vi "returnState.vi"(6 "error IN":errorcluster, 8 "String IN":string) -> (0 "error out":errorcluster, 1 "Return State":T2(ring), 3 "output cluster":T1)   [LabVIEW 2017]
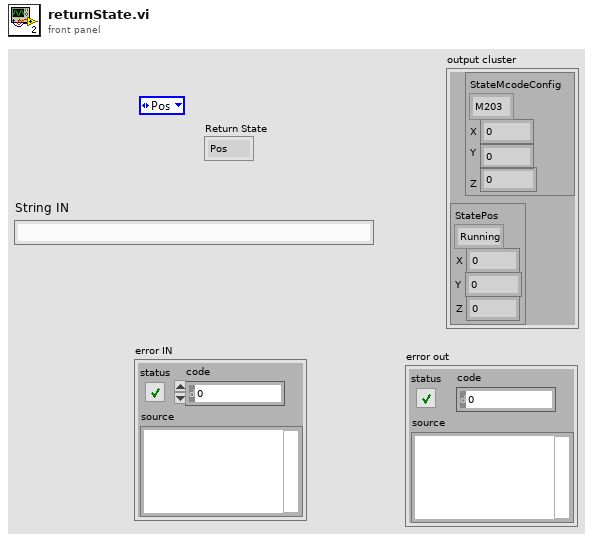
[diagram p1: front panel]
types:
  T1 = cluster{"OUTCONFIG":cluster{"StateMcodeConfig":enum16{"M203", "M201", "M92", "M3001"}, "X":dbl, "Y":dbl, "Z":dbl}, "outPOS":cluster{"StatePos":enum16{"Running", "Waiting", "Pos", "IDLE"}, "X":dbl, "Z":dbl, "Y":dbl}}
  T2 = enum16{"Pos", "Config", "Data1", "Data2", "Step"}
  T3 = cluster{"Enum":enum16{"Running", "Waiting", "Pos", "IDLE"}, dbl, dbl, dbl}
  T4 = cluster{"StateMcodeConfig":enum16{"M203", "M201", "M92", "M3001"}, dbl, dbl, dbl}
  T5 = cluster{cluster{"StateMcodeConfig":enum16{"M203", "M201", "M92", "M3001"}, dbl, dbl, dbl}, cluster{"Enum":enum16{"Running", "Waiting", "Pos", "IDLE"}, dbl, dbl, dbl}}
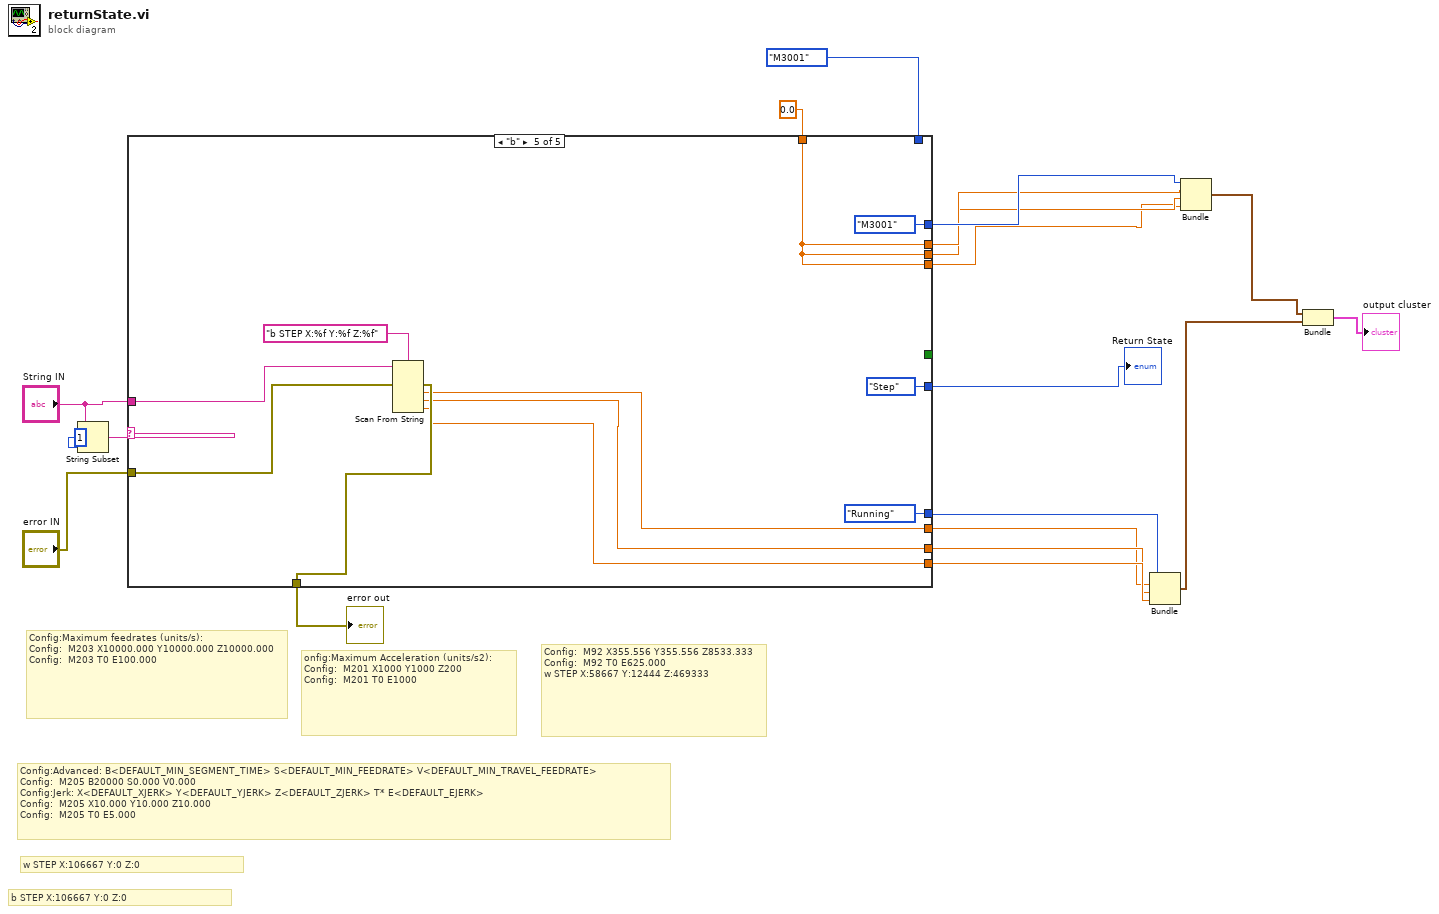
[diagram p0: block diagram]
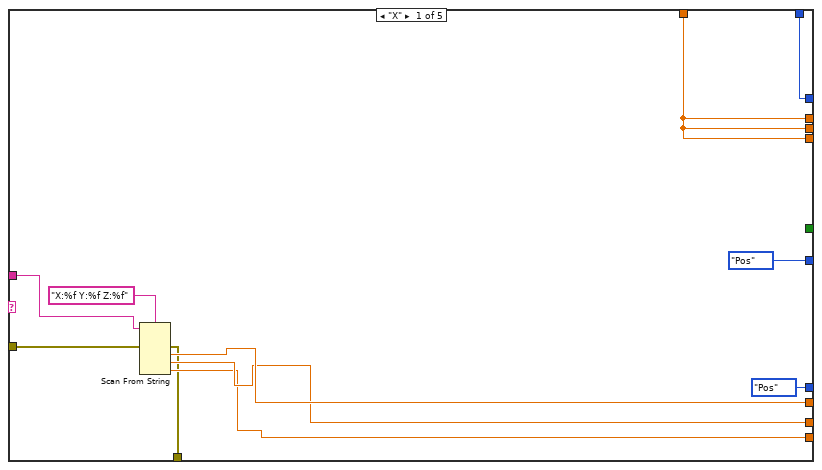
[diagram p2: hidden frame]
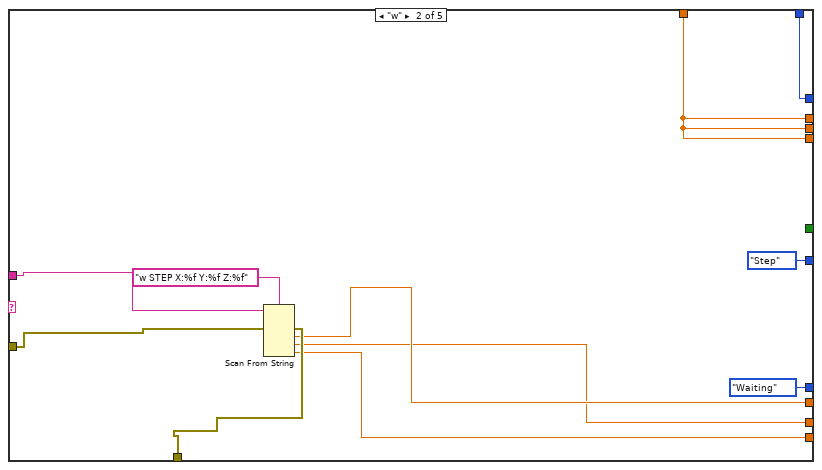
[diagram p3: hidden frame]
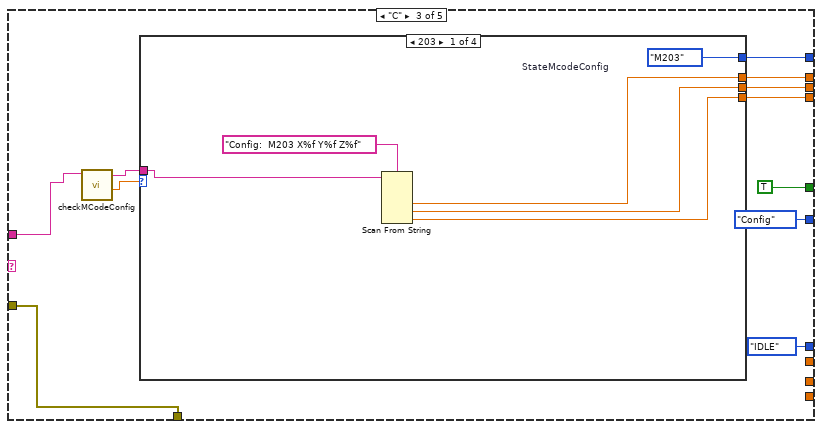
[diagram p4: hidden frame]
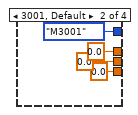
[diagram p5: hidden frame]
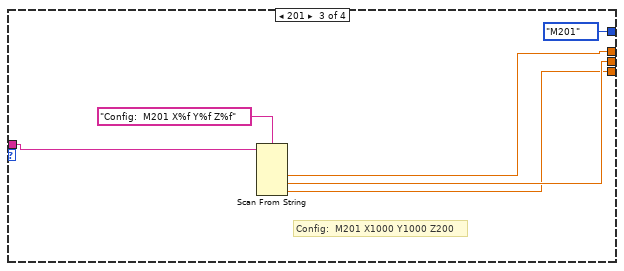
[diagram p6: hidden frame]
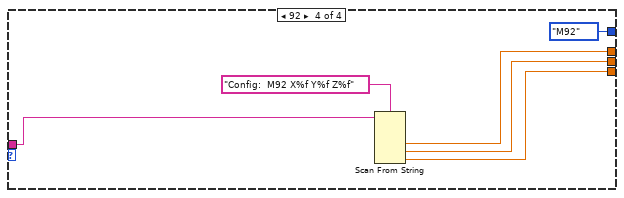
[diagram p7: hidden frame]
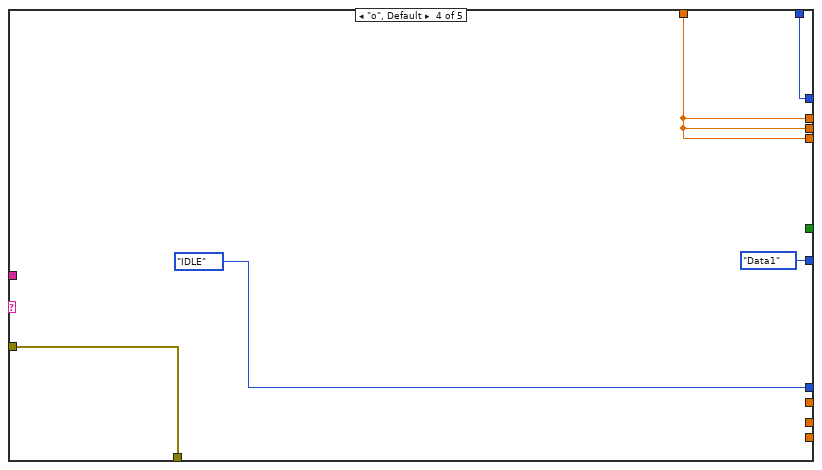
[diagram p8: hidden frame]
diagram:
  # "b STEP X:106667 Y:0 Z:0"
  # "Config:Advanced: B<DEFAULT_MIN_SEGMENT_TIME> S<DEFAULT_MIN_FEEDRATE> V<DEFAULT_MIN_TRAVEL_FEEDRATE>\nConfig:  M205 B20000 S0.000 V0.000\nConfig:Jerk: X<DEFAULT_XJERK> Y<DEFAULT_YJERK> Z<DEFAULT_ZJERK> T* E<DEFAULT_EJERK>\nConfig:  M205 X10.000 Y10.000 Z10.000\nConfig:  M205 T0 E5.000"
  # "Config:  M92 X355.556 Y355.556 Z8533.333\nConfig:  M92 T0 E625.000\nw STEP X:58667 Y:12444 Z:469333"
  # "onfig:Maximum Acceleration (units/s2):\nConfig:  M201 X1000 Y1000 Z200\nConfig:  M201 T0 E1000"
  # "Config:Maximum feedrates (units/s):\nConfig:  M203 X10000.000 Y10000.000 Z10000.000\nConfig:  M203 T0 E100.000"
  # "w STEP X:106667 Y:0 Z:0"
  n1 = String Subset(string="String IN", length (rest)=1 ("length (rest)")) -> (substring=w18:string)  [unwired: 1 in]
  n2 = case shown="\"b\"" w18 {
    tunnel: [enum16{"Running", "Waiting", "Pos", "IDLE"}."Pos" ("Enum") enum16{"Running", "Waiting", "Pos", "IDLE"}."Waiting" ("Enum") enum16{"Running", "Waiting", "Pos", "IDLE"}."IDLE" ("Enum") enum16{"Running", "Waiting", "Pos", "IDLE"}."IDLE" ("Enum") enum16{"Running", "Waiting", "Pos", "IDLE"}."Running" ("Enum")] -> w14
    tunnel: "String IN" -> [w29 w40 w50 _ w86]
    tunnel: [w28 w37 _ _ w83] -> w11
    tunnel: [w27 w36 _ _ w82] -> w12
    tunnel: [w26 w33 _ _ w81] -> w13
    tunnel: "error IN" -> [w25 w39 w52 w78 w85]
    tunnel: [w24 w38 w52 w78 w84] -> w15
    tunnel: [w23 w34 w47 w76 w89] -> w7
    tunnel: [w23 w34 w46 w76 w89] -> w6
    tunnel: [w23 w34 w45 w76 w89] -> w5
    tunnel: [w21 w35 w44 w77 enum16{"M203", "M201", "M92", "M3001"}."M3001" ("StateMcodeConfig")] -> w8
    tunnel: enum16{"M203", "M201", "M92", "M3001"}."M3001" ("StateMcodeConfig") -> [w21 w35 _ w77 _]
    tunnel: 0.0 -> [w23 w34 _ w76 w89]
    tunnel: [_ _ TRUE ("Status") _ _] -> _
    tunnel: [T2."Pos" ("Return State") T2."Step" ("Return State") T2."Config" ("Return State") T2."Data1" ("Return State") T2."Step" ("Return State")] -> w4
    frame "X" {
      n3 = Scan From String(format string="X:%f Y:%f Z:%f", input string=w29, error in=w25) -> (error out=w24:errorcluster, output 1=w28:dbl, output 2=w27:dbl, output 3=w26:dbl)  [unwired: 4 in, 2 out]
    }
    frame "w" {
      n4 = Scan From String(format string="w STEP X:%f Y:%f Z:%f", input string=w40, error in=w39) -> (error out=w38:errorcluster, output 1=w37:dbl, output 2=w36:dbl, output 3=w33:dbl)  [unwired: 4 in, 2 out]
    }
    frame "C" {
      n5 = call "checkMCodeConfig.vi"("INPUT"=w50) -> ("MCODE"=w49:dbl, "OUTPUT"=w48:string)  [unwired: 9 in]
      n6 = case shown="203" w49 {
        tunnel: w48 -> [w57 _ w67 w73]
        tunnel: [w56 0.0 w66 w72] -> w47
        tunnel: [w55 0.0 w65 w71] -> w46
        tunnel: [w54 0.0 w64 w70] -> w45
        tunnel: [w53 enum16{"M203", "M201", "M92", "M3001"}."M3001" ("StateMcodeConfig") enum16{"M203", "M201", "M92", "M3001"}."M201" ("StateMcodeConfig") enum16{"M203", "M201", "M92", "M3001"}."M92" ("StateMcodeConfig")] -> w44
        frame 203 {
          w53 = enum16{"M203", "M201", "M92", "M3001"}."M203"  # StateMcodeConfig
          n7 = Scan From String(format string="Config:  M203 X%f Y%f Z%f", input string=w57) -> (output 1=w56:dbl, output 2=w55:dbl, output 3=w54:dbl)  [unwired: 5 in, 3 out]
        }
        frame 3001, Default {
        }
        frame 201 {
          # "Config:  M201 X1000 Y1000 Z200"
          n8 = Scan From String(format string="Config:  M201 X%f Y%f Z%f", input string=w67) -> (output 1=w66:dbl, output 2=w65:dbl, output 3=w64:dbl)  [unwired: 5 in, 3 out]
        }
        frame 92 {
          n9 = Scan From String(format string="Config:  M92 X%f Y%f Z%f", input string=w73) -> (output 1=w72:dbl, output 2=w71:dbl, output 3=w70:dbl)  [unwired: 5 in, 3 out]
        }
      }
    }
    frame "o", Default {
    }
    frame "b" {
      n10 = Scan From String(format string="b STEP X:%f Y:%f Z:%f", input string=w86, error in=w85) -> (error out=w84:errorcluster, output 1=w83:dbl, output 2=w82:dbl, output 3=w81:dbl)  [unwired: 4 in, 2 out]
    }
  }
  "error out" <- w15
  "Return State" <- w4
  n11 = Bundle("Enum"=w14, w11, w12, w13) -> (w2:T3)  [unwired: 1 in]
  n12 = Bundle("StateMcodeConfig"=w8, w7, w6, w5) -> (w1:T4)  [unwired: 1 in]
  n13 = Bundle(w1, w2) -> (→"output cluster":T5)  [unwired: 1 in]
